vi "binary record both ch_v01.vi"(4 "Record":bool, 7 "Files path array":path[](array[path]), 8 "reference":refnum<vi>, 10 "wfm":i16[][](array[numeric]), 11 "Chan 1 params":T1) -> ()   [LabVIEW 2013]
panel:
  out "error out":errorcluster
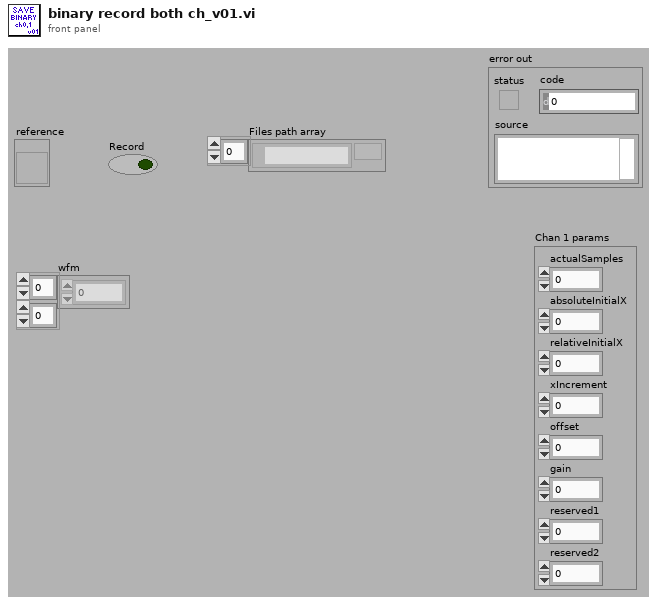
[diagram p1: front panel]
types:
  T1 = cluster{"actualSamples":i32, "absoluteInitialX":dbl, "relativeInitialX":dbl, "xIncrement":dbl, "offset":dbl, "gain":dbl, "reserved1":dbl, "reserved2":dbl}
  T2 = enum16{"open", "replace", "create", "open or create", "replace or create", "replace or create with confirmation"}
  T3 = enum16{"big-endian, network order", "native, host order", "little-endian"}
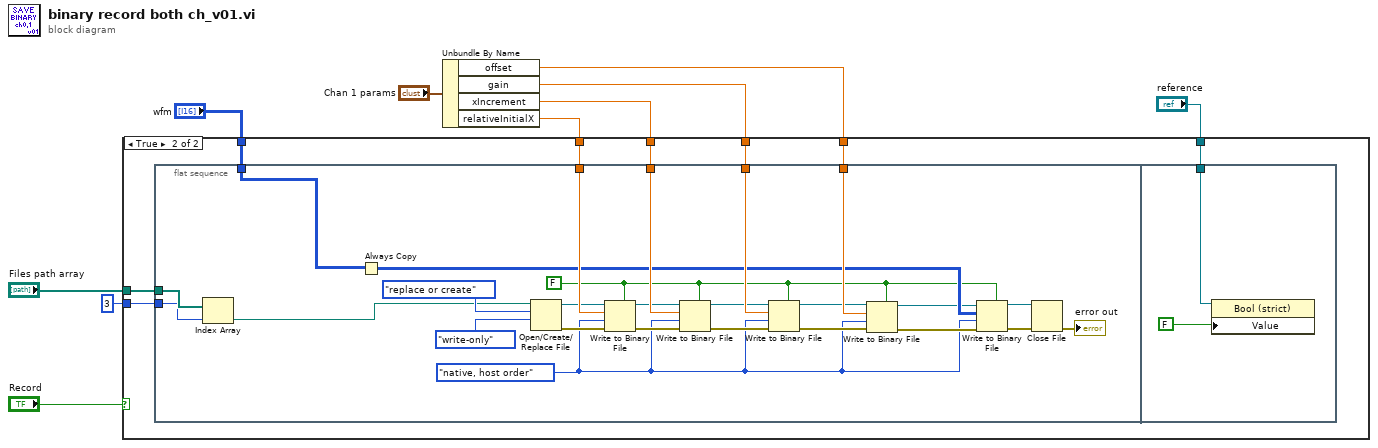
[diagram p0: block diagram]
diagram:
  n1 = Unbundle By Name("Chan 1 params") -> ("offset"=w1:dbl, "gain"=w2:dbl, "xIncrement"=w3:dbl, "relativeInitialX"=w4:dbl)
  n2 = case shown="True" "Record" {
    tunnel: "wfm" -> [_ w18]
    tunnel: w4 -> [_ w17]
    tunnel: w3 -> [_ w16]
    tunnel: w2 -> [_ w15]
    tunnel: w1 -> [_ w14]
    tunnel: "reference" -> [_ w13]
    tunnel: "Files path array" -> [_ w12]
    tunnel: 3 ("Index files\npath array") -> [_ w11]
    frame False {
    }
    frame True {
      n3 = flat-sequence {
        tunnel: w18 -> [w20]
        tunnel: w17 -> [w44]
        tunnel: w16 -> [w43]
        tunnel: w15 -> [w42]
        tunnel: w14 -> [w41]
        tunnel: w12 -> [w22]
        tunnel: w11 -> [w21]
        tunnel: w13 -> [w45]
        frame #0 {
          w24 = FALSE ("prepend array or string size? (T)")
          w25 = T3."native, host order" ("byte order (0:big-endian, network order)")
          n4 = Index Array(array=w22, index=w21) -> (element=w23:path)
          n5 = Always Copy(1:w20) -> (0:w38:i16[][])
          n6 = Open/Create/Replace File(file path (use dialog)=w23, operation (0:open)=T2."replace or create", access (0:read/write)=enum16{"read/write", "read-only", "write-only"}."write-only") -> (refnum out=w37:refnum<file>, error out=w36:errorcluster)  [unwired: 1 in, 3 out]
          n7 = Write to Binary File(file (use dialog)=w37, data=w44, error in=w36, 5:w24, 9:w25) -> (refnum out=w35:refnum<file>, error out=w34:errorcluster)  [unwired: 2 out]
          n8 = Write to Binary File(file (use dialog)=w35, data=w43, error in=w34, 5:w24, 9:w25) -> (refnum out=w33:refnum<file>, error out=w29:errorcluster)  [unwired: 2 out]
          n9 = Write to Binary File(file (use dialog)=w33, data=w42, error in=w29, 5:w24, 9:w25) -> (refnum out=w32:refnum<file>, error out=w28:errorcluster)  [unwired: 2 out]
          n10 = Write to Binary File(file (use dialog)=w32, data=w41, error in=w28, 5:w24, 9:w25) -> (refnum out=w31:refnum<file>, error out=w27:errorcluster)  [unwired: 2 out]
          n11 = Write to Binary File(file (use dialog)=w31, data=w38, error in=w27, 5:w24, 9:w25) -> (refnum out=w30:refnum<file>, error out=w26:errorcluster)  [unwired: 2 out]
          n12 = Close File(refnum=w30, error in=w26) -> (error out=→"error out":errorcluster)  [unwired: 1 out]
        }
        frame #1 {
          n13 = property on="Property Node" class="Bool (strict)"(reference=w45, "Value"=FALSE ("Boolean")) -> ()  [unwired: 1 in, 2 out]
        }
      }
    }
  }
